vi "fiberphotometry_liveview.vi"() -> ()   [LabVIEW 2020]
uses:
  <userlib>/AndorSDK3/Data/GetPixelData16.vi
panel:
  in  "AOI Top":i64
  in  "AOI Left":i64
  in  "Binning":string
  in  "405 nm power (%)":i32
  in  "470 nm power (%)":i32
  in  "Apply Settings":bool
  in  "Centre AOI":bool
  in  "AOI Width":i64
  in  "AOI Height":i64
  out "Ready":bool
  in  "Run":bool
  in  "error":errorcluster
  out "Pixel Encoding":string
  out "Intensity Graph":u16[][](graph)
  out "AOIStride":i64
  out "PixelData":u16[](array[numeric])
  out "ByteData":u8[](array[numeric])
  in  "ExposureTime":dbl=0.1
  out "ImageSizeBytes":i64
  out "Handle":i32
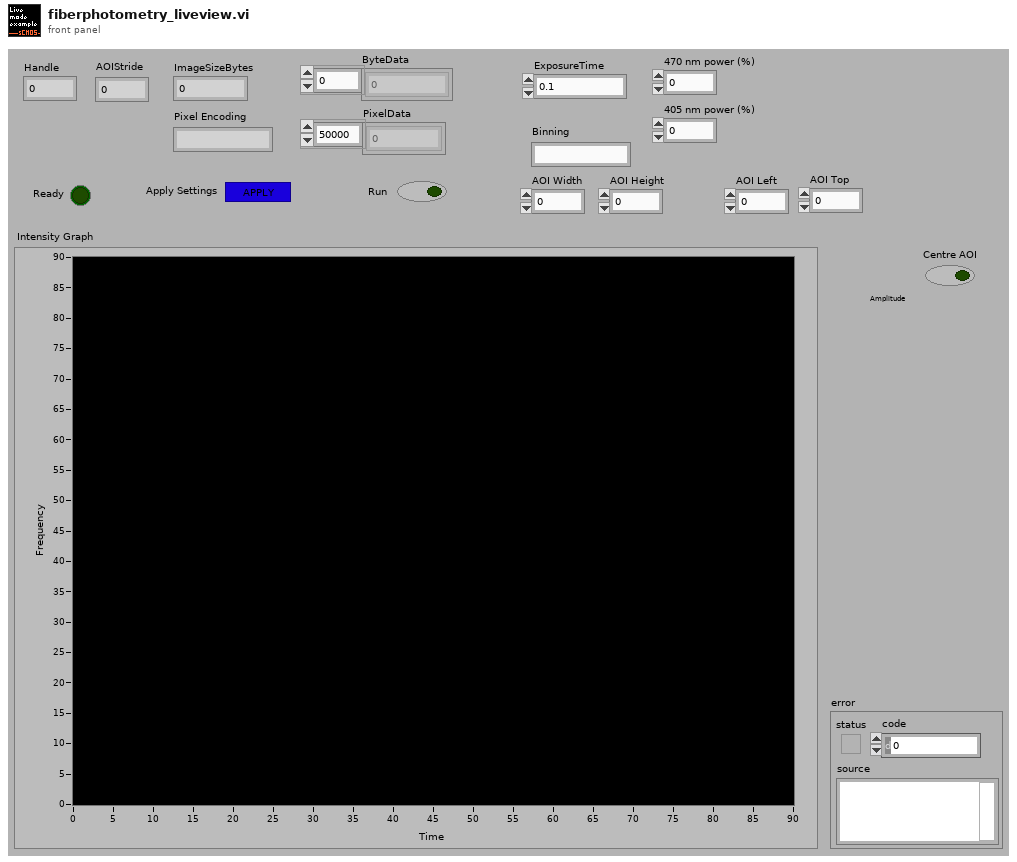
[diagram p1: front panel]
types:
  T1 = enum8{"Enabled", "Disabled", "Disabled and Grayed Out"}
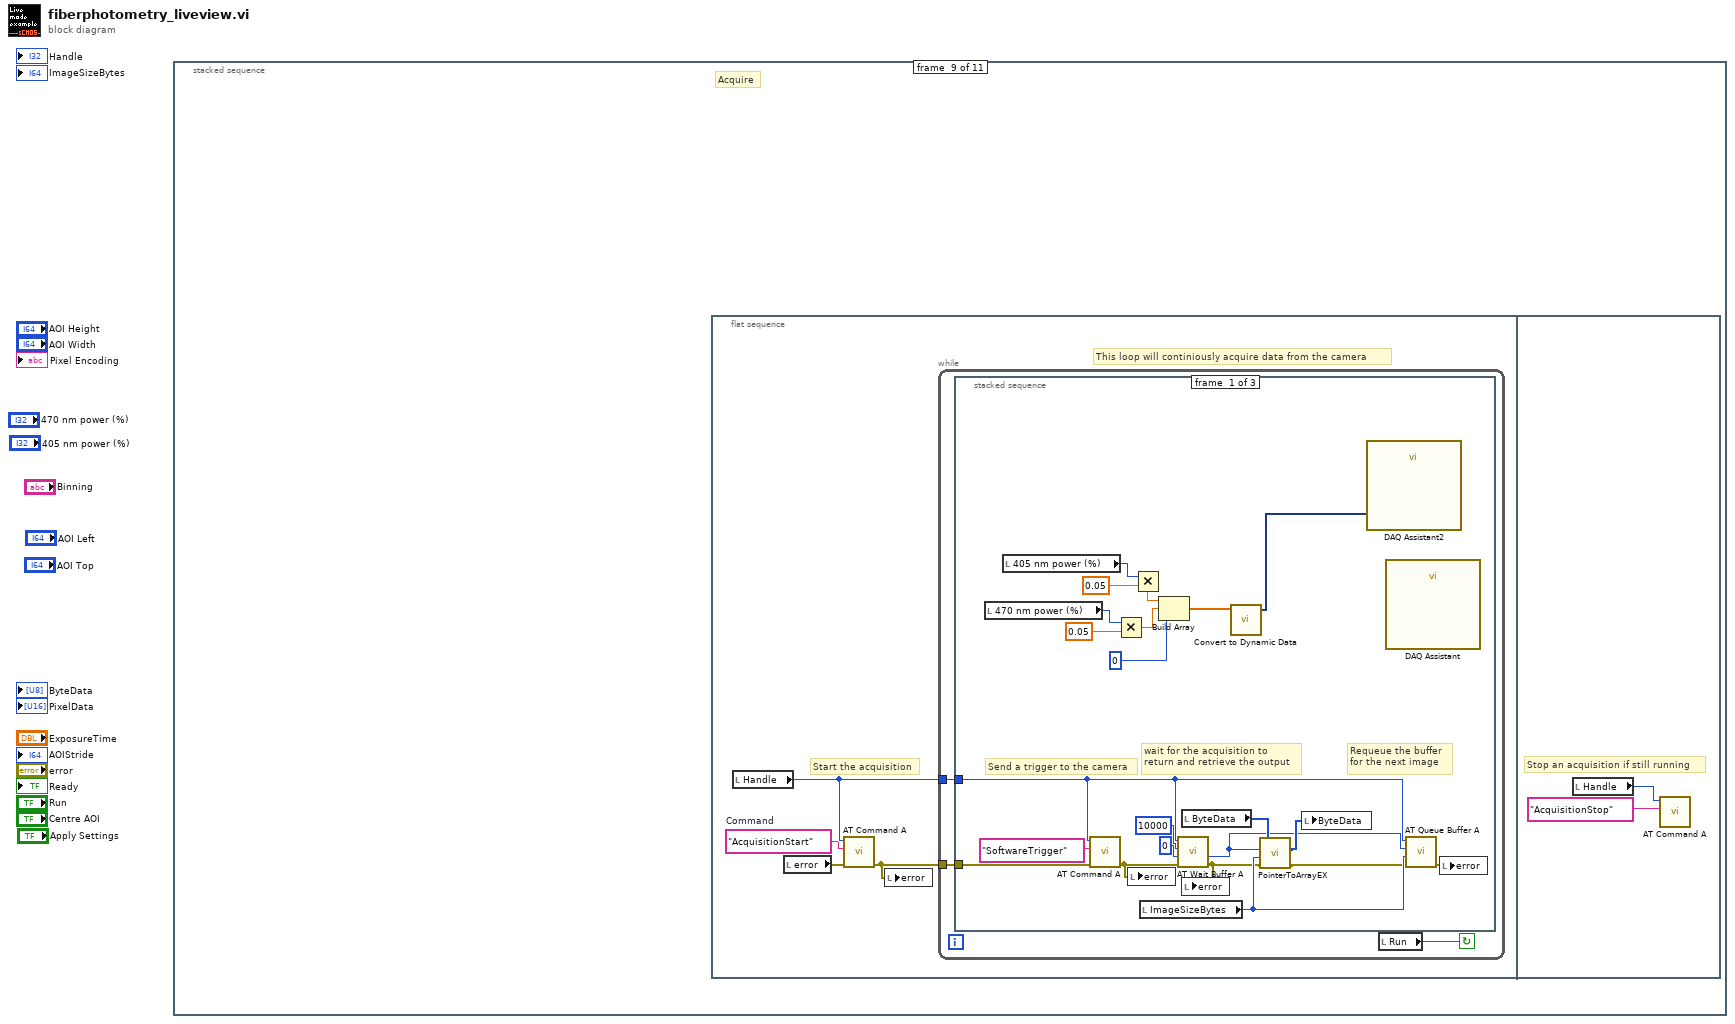
[diagram p0: block diagram]
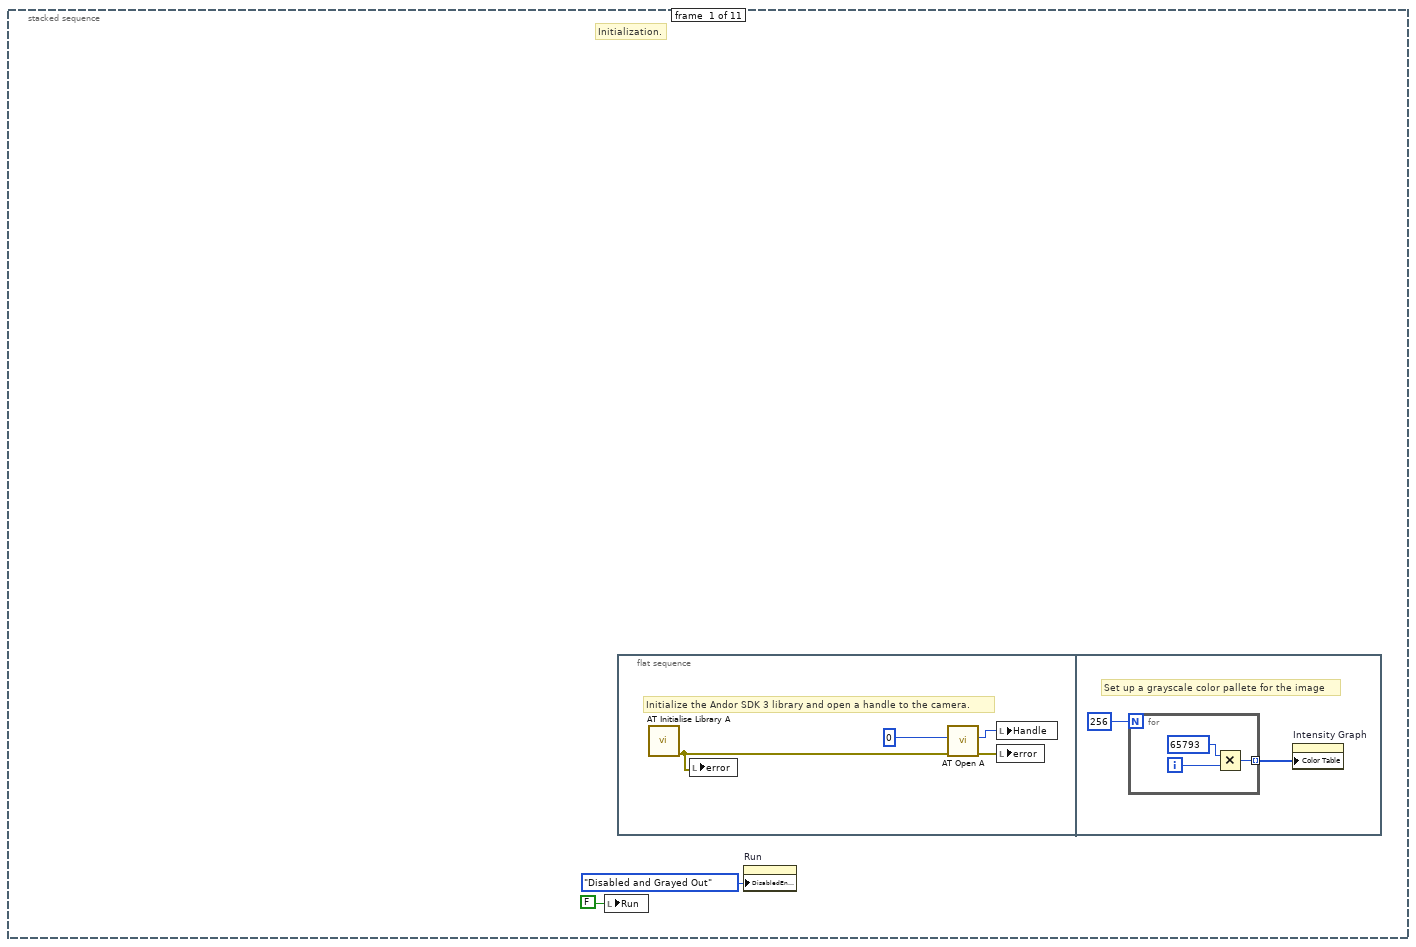
[diagram p2: hidden frame]
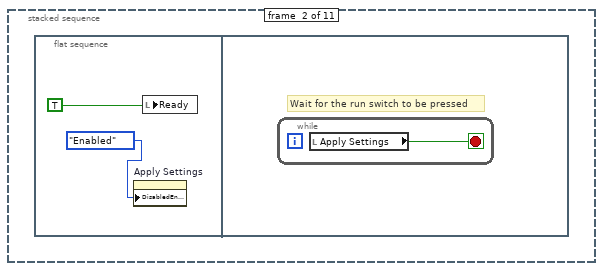
[diagram p3: hidden frame]
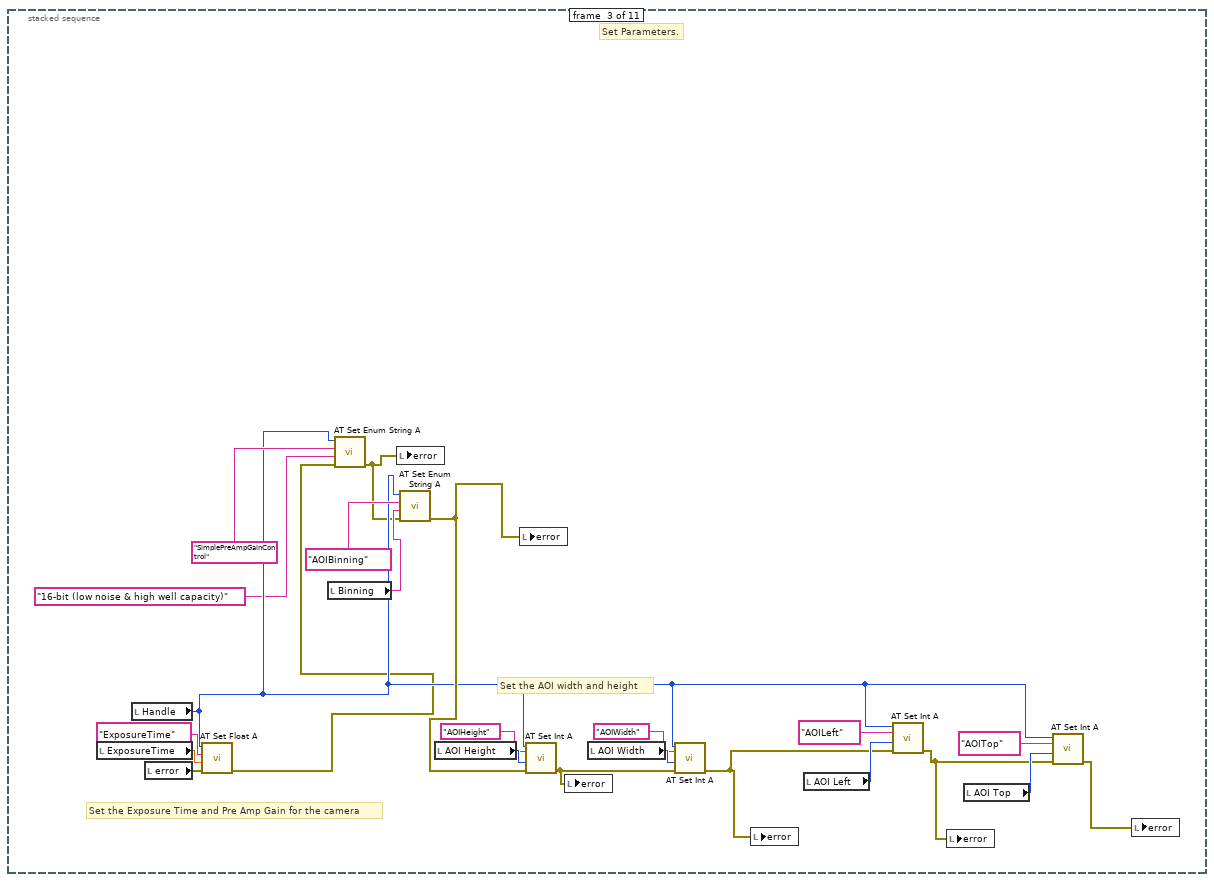
[diagram p4: hidden frame]
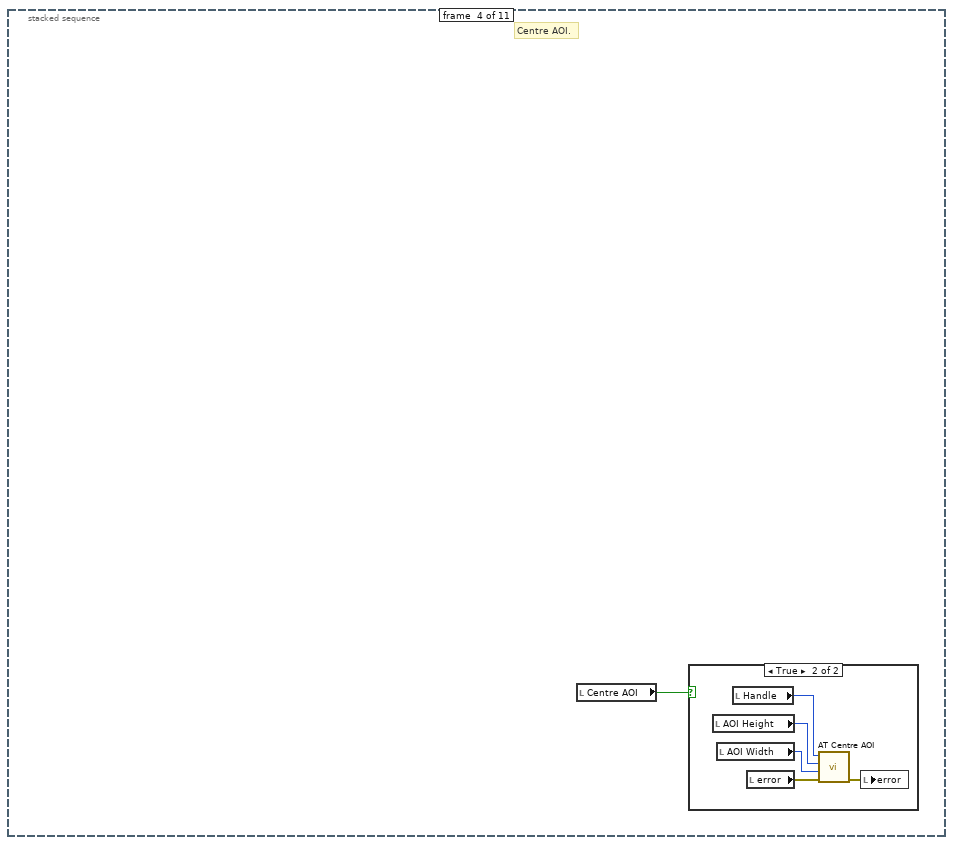
[diagram p5: hidden frame]
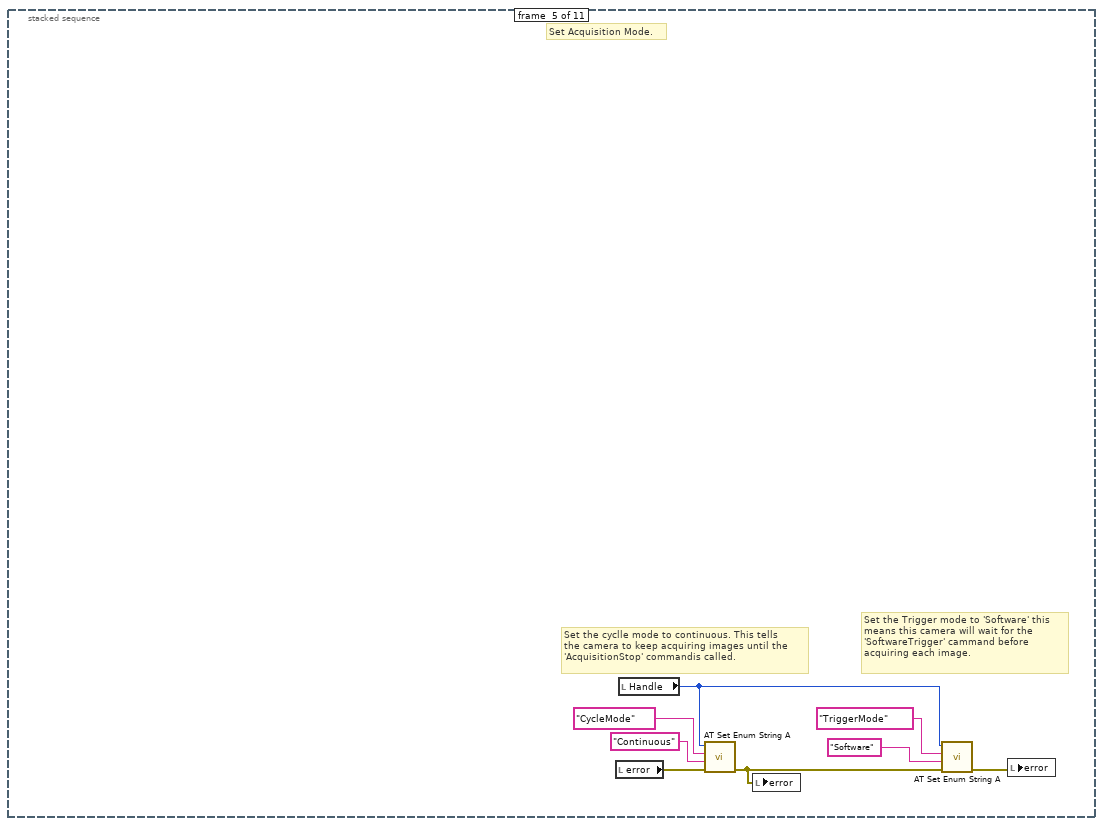
[diagram p7: hidden frame]
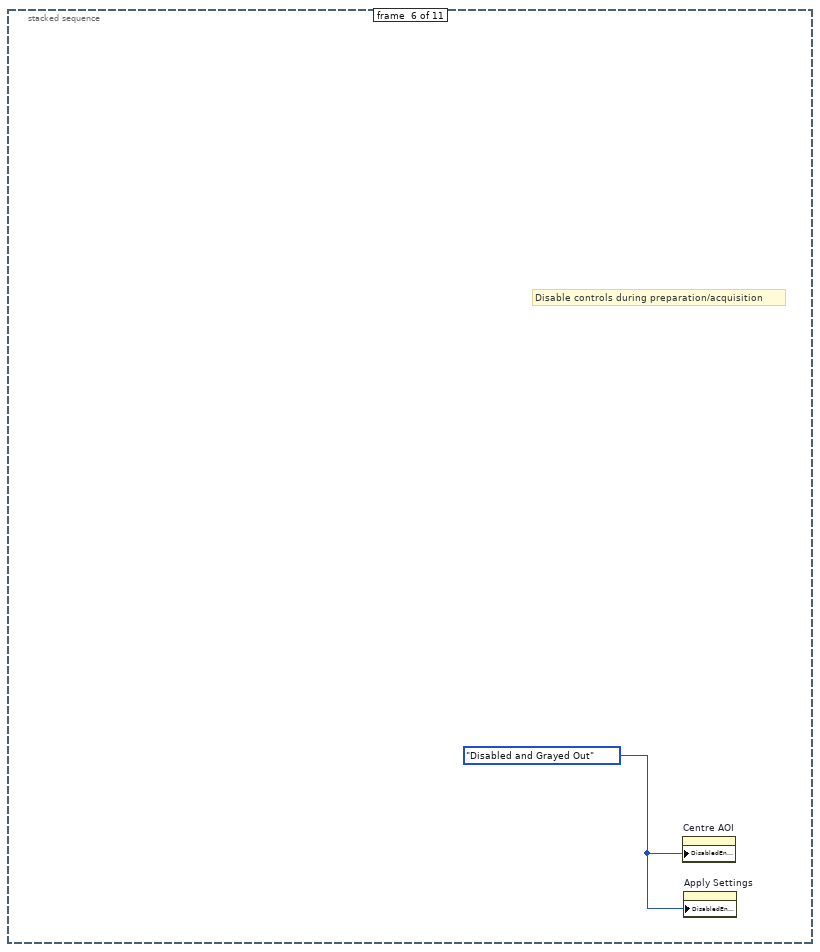
[diagram p8: hidden frame]
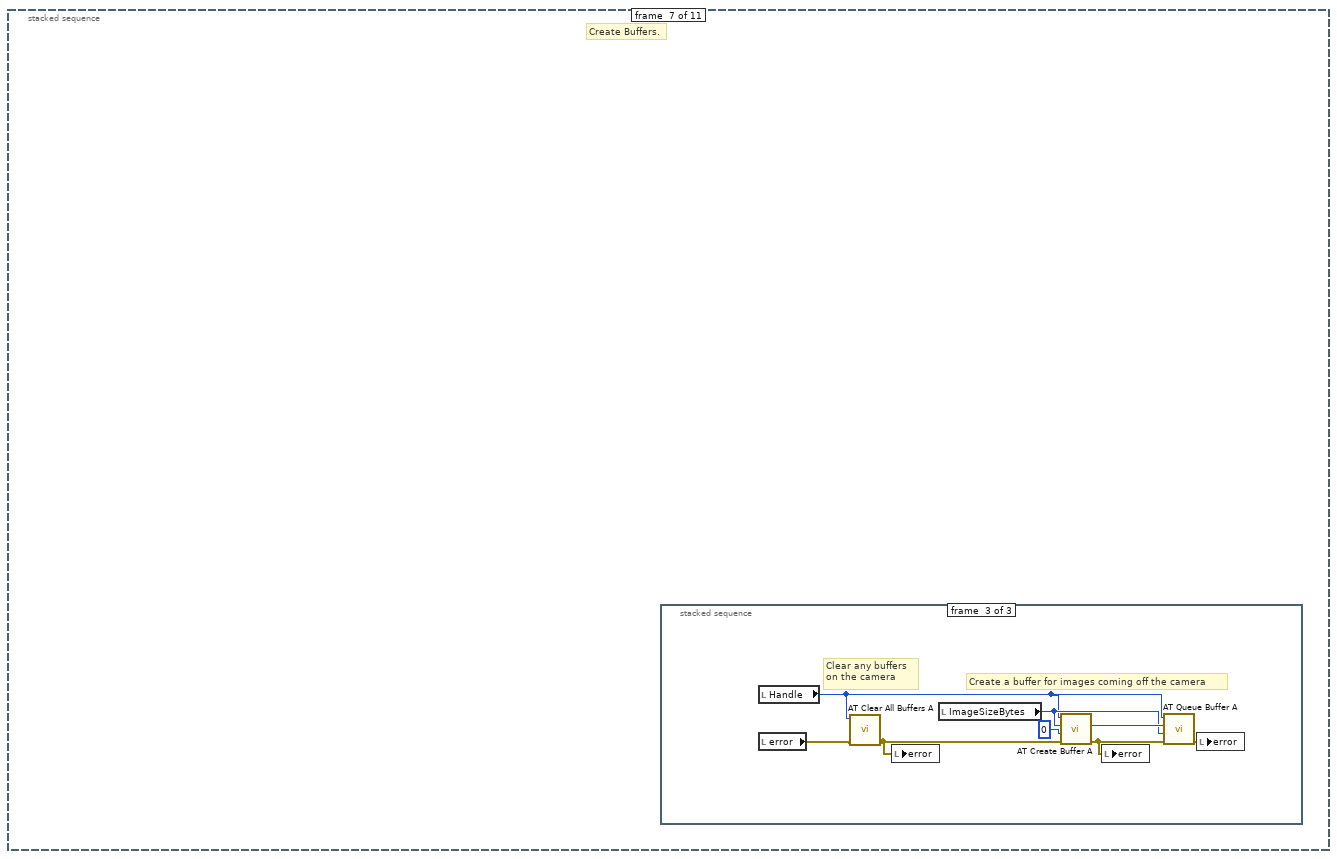
[diagram p9: hidden frame]
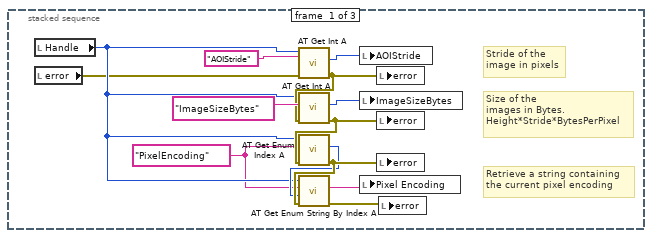
[diagram p10: hidden frame]
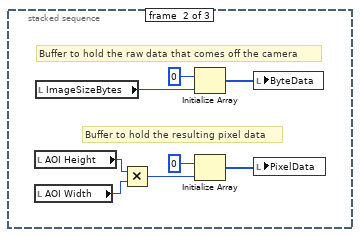
[diagram p11: hidden frame]
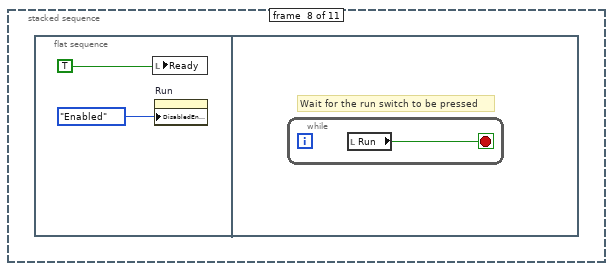
[diagram p12: hidden frame]
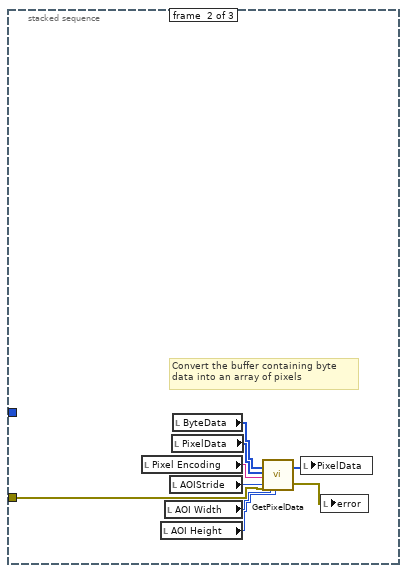
[diagram p13: hidden frame]
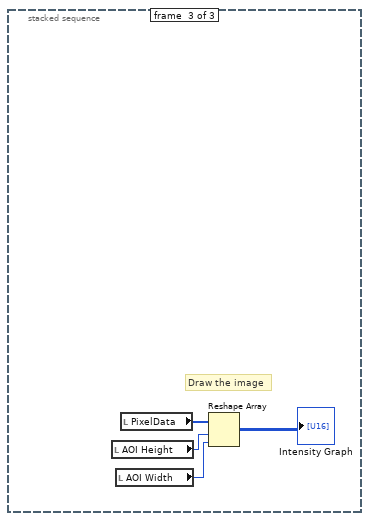
[diagram p14: hidden frame]
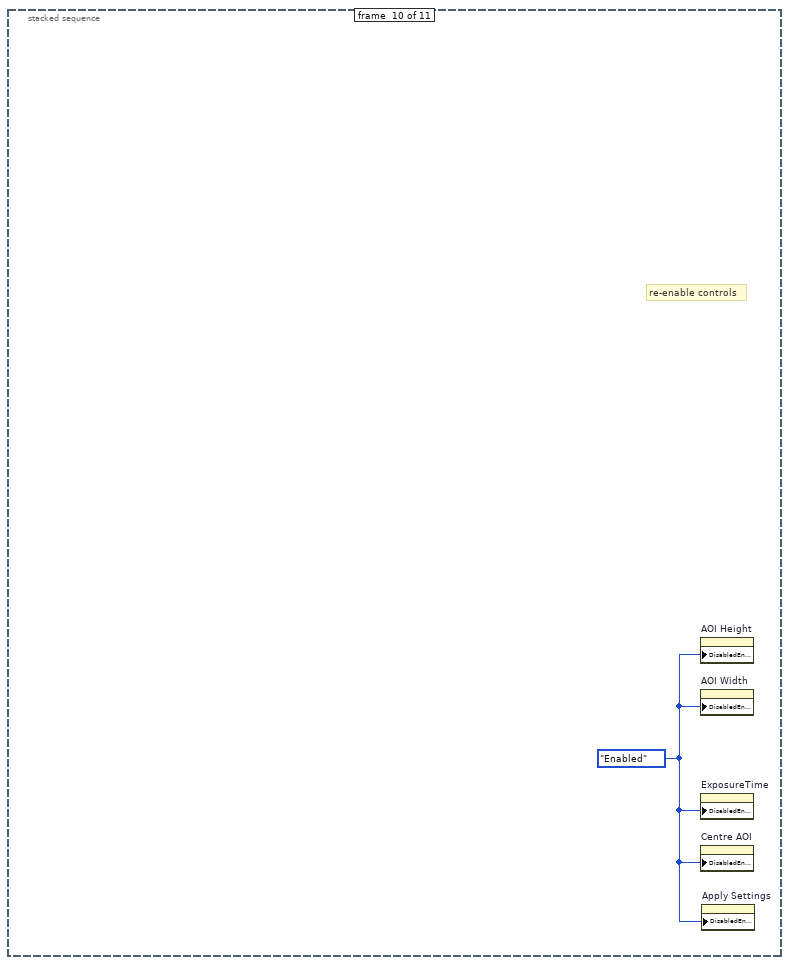
[diagram p15: hidden frame]
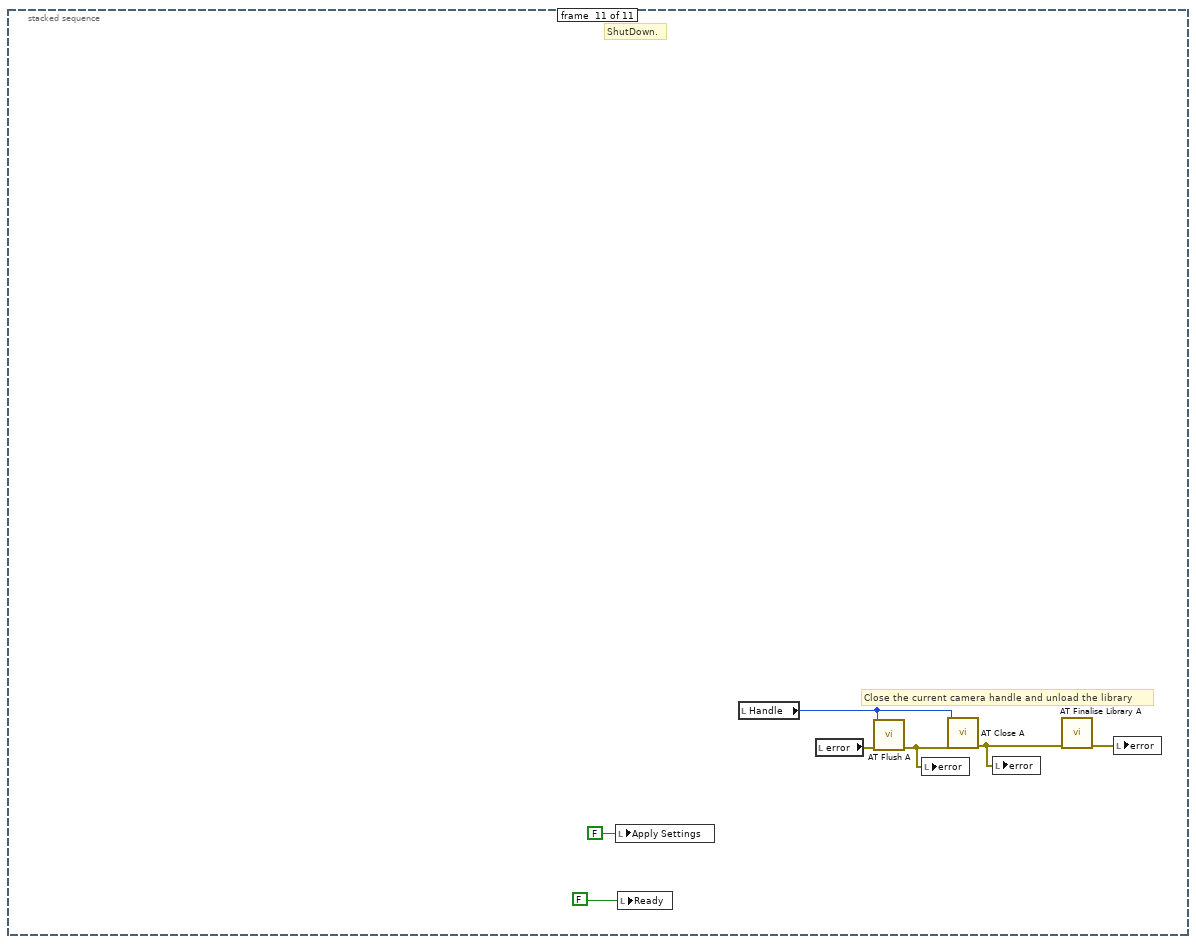
[diagram p16: hidden frame]
diagram:
  n1 = stacked-sequence {
    frame #0 {
      # "Initialization."
      n2 = local write "Run"(FALSE ("Run")) -> ()
      n3 = flat-sequence {
        frame #0 {
          # "Initialize the Andor SDK 3 library and open a handle to the camera."
          n4 = call <userlib>:"AT Initialise Library A.vi"() -> ("error out"=w4:errorcluster)  [unwired: 10 in, 1 out]
          n5 = local write "error"(w4) -> ()
          n6 = call <userlib>:"AT Open A.vi"("error in (no error)"=w4, "CameraIndex"=0) -> ("error out"=w3:errorcluster, "Handle"=w5:i32)  [unwired: 7 in, 1 out]
          n7 = local write "Handle"(w5) -> ()
          n8 = local write "error"(w3) -> ()
        }
        frame #1 {
          # "Set up a grayscale color pallete for the image"
          n9 = for {
            N: 256 -> [_]
            tunnel: [w10] -> w7 mode=indexing
            i -> [w11]
            n10 = Multiply(x=65793, y=w11) -> (x*y=w10:i32)
          }
          n11 = property on="Intensity Graph" class="IntGraph (strict)"("Color Table"=w7) -> ()  [unwired: 2 in, 2 out]
        }
      }
      n12 = property on="Run" class="Bool (strict)"("DisabledEnum"=T1."Disabled and Grayed Out" ("Disabled")) -> ()  [unwired: 2 in, 2 out]
    }
    frame #1 {
      n13 = flat-sequence {
        frame #0 {
          n14 = property on="Apply Settings" class="Bool (strict)"("DisabledEnum"=T1."Enabled" ("Disabled")) -> ()  [unwired: 2 in, 2 out]
          n15 = local write "Ready"(TRUE ("Ready")) -> ()
        }
        frame #1 {
          # "Wait for the run switch to be pressed"
          n16 = while {
            stop <- w14 stop-if-true
            n17 = local read "Apply Settings"() -> (w14:bool)
          }
        }
      }
    }
    frame #2 {
      # "Set the AOI width and height"
      # "Set the Exposure Time and Pre Amp Gain for the camera"
      # "Set Parameters."
      n18 = local read "ExposureTime"() -> (w37:dbl)
      n19 = local read "Handle"() -> (w18:i32)
      n20 = local read "error"() -> (w35:errorcluster)
      n21 = call <userlib>:"AT Set Float A.vi"("error in (no error)"=w35, "Value"=w37, "Feature"="ExposureTime" ("ExposureTime"), "Hndl"=w18) -> ("error out"=w17:errorcluster)  [unwired: 6 in, 1 out]
      n22 = local read "Binning"() -> (w28:string)
      n23 = call <userlib>:"AT Set Enum String A.vi"("error in (no error)"=w17, "String"="16-bit (low noise & high well capacity)", "Feature"="SimplePreAmpGainControl" ("Enum feature"), "Handle"=w18) -> ("error out"=w16:errorcluster)  [unwired: 6 in, 1 out]
      n24 = local write "error"(w16) -> ()
      n25 = call <userlib>:"AT Set Enum String A.vi"("error in (no error)"=w16, "String"=w28, "Feature"="AOIBinning" ("Enum feature"), "Handle"=w18) -> ("error out"=w27:errorcluster)  [unwired: 6 in, 1 out]
      n26 = local read "AOI Height"() -> (w33:i64)
      n27 = local write "error"(w27) -> ()
      n28 = call <userlib>:"AT Set Int A.vi"("error in (no error)"=w27, "Value"=w33, "Feature"="AOIHeight" ("Integer feature"), "Handle"=w18) -> ("error out"=w34:errorcluster)  [unwired: 6 in, 1 out]
      n29 = local write "error"(w34) -> ()
      n30 = local read "AOI Width"() -> (w32:i64)
      n31 = call <userlib>:"AT Set Int A.vi"("error in (no error)"=w34, "Value"=w32, "Feature"="AOIWidth" ("Integer feature 2"), "Handle"=w18) -> ("error out"=w22:errorcluster)  [unwired: 6 in, 1 out]
      n32 = local write "error"(w22) -> ()
      n33 = local read "AOI Left"() -> (w26:i64)
      n34 = call <userlib>:"AT Set Int A.vi"("error in (no error)"=w22, "Value"=w26, "Feature"="AOILeft" ("Integer feature 2"), "Handle"=w18) -> ("error out"=w21:errorcluster)  [unwired: 6 in, 1 out]
      n35 = local write "error"(w21) -> ()
      n36 = local read "AOI Top"() -> (w24:i64)
      n37 = call <userlib>:"AT Set Int A.vi"("error in (no error)"=w21, "Value"=w24, "Feature"="AOITop" ("Integer feature 2"), "Handle"=w18) -> ("error out"=w20:errorcluster)  [unwired: 6 in, 1 out]
      n38 = local write "error"(w20) -> ()
    }
    frame #3 {
      # "Centre AOI."
      n39 = local read "Centre AOI"() -> (w38:bool)
      n40 = case shown="True" w38 {
        frame False {
        }
        frame True {
          n41 = local read "AOI Height"() -> (w40:i64)
          n42 = local read "AOI Width"() -> (w41:i64)
          n43 = local read "Handle"() -> (w39:i32)
          n44 = local read "error"() -> (w42:errorcluster)
          n45 = call <userlib>:"AT Centre AOI.vi"("error in (no error)"=w42, "AOI Width"=w41, "AOI Height"=w40, "Handle"=w39) -> ("error out"=w43:errorcluster)  [unwired: 7 in]
          n46 = local write "error"(w43) -> ()
        }
      }
    }
    frame #4 {
      # "Set the Trigger mode to 'Software' this \nmeans this camera will wait for the \n'SoftwareTrigger' cammand before \nacquiring each image."
      # "Set the cyclle mode to continuous. This tells \nthe camera to keep acquiring images until the \n'AcquisitionStop' commandis called."
      # "Set Acquisition Mode."
      n47 = local read "error"() -> (w50:errorcluster)
      n48 = local read "Handle"() -> (w48:i32)
      n49 = call <userlib>:"AT Set Enum String A.vi"("error in (no error)"=w50, "String"="Continuous", "Feature"="CycleMode" ("Enum feature"), "Handle"=w48) -> ("error out"=w49:errorcluster)  [unwired: 6 in, 1 out]
      n50 = local write "error"(w49) -> ()
      n51 = call <userlib>:"AT Set Enum String A.vi"("error in (no error)"=w49, "String"="Software", "Feature"="TriggerMode" ("Enum feature"), "Handle"=w48) -> ("error out"=w46:errorcluster)  [unwired: 6 in, 1 out]
      n52 = local write "error"(w46) -> ()
    }
    frame #5 {
      w52 = T1."Disabled and Grayed Out" ("Disabled")
      # "Disable controls during preparation/acquisition"
      n53 = property on="Centre AOI" class="Bool (strict)"("DisabledEnum"=w52) -> ()  [unwired: 2 in, 2 out]
      n54 = property on="Apply Settings" class="Bool (strict)"("DisabledEnum"=w52) -> ()  [unwired: 2 in, 2 out]
    }
    frame #6 {
      # "Create Buffers."
      n55 = stacked-sequence {
        frame #0 {
          w53 = "PixelEncoding" ("Enum feature")
          # "Retrieve a string containing \nthe current pixel encoding"
          # "Stride of the\nimage in pixels"
          # "Size of the\nimages in Bytes.\nHeight*Stride*BytesPerPixel"
          n56 = local read "Handle"() -> (w55:i32)
          n57 = local read "error"() -> (w54:errorcluster)
          n58 = call <userlib>:"AT Get Int A.vi"("error in (no error)"=w54, "Feature"="AOIStride" ("Integer feature"), "Handle"=w55) -> ("error out"=w61:errorcluster, "Value"=w65:i64)  [unwired: 6 in, 1 out]
          n59 = call <userlib>:"AT Get Int A.vi"("error in (no error)"=w61, "Feature"="ImageSizeBytes" ("Integer feature"), "Handle"=w55) -> ("error out"=w60:errorcluster, "Value"=w64:i64)  [unwired: 6 in, 1 out]
          n60 = call <userlib>:"AT Get Enum Index A.vi"("error in (no error)"=w60, "Feature"=w53, "Handle"=w55) -> ("error out"=w59:errorcluster, "Value"=w58:i32)  [unwired: 6 in, 1 out]
          n61 = call <userlib>:"AT Get Enum String By Index A.vi"("error in (no error)"=w59, "Index"=w58, "Feature"=w53, "Handle"=w55) -> ("error out"=w56:errorcluster, "String"=w57:string)  [unwired: 5 in, 1 out]
          n62 = local write "AOIStride"(w65) -> ()
          n63 = local write "ImageSizeBytes"(w64) -> ()
          n64 = local write "Pixel Encoding"(w57) -> ()
          n65 = local write "error"(w61) -> ()
          n66 = local write "error"(w60) -> ()
          n67 = local write "error"(w59) -> ()
          n68 = local write "error"(w56) -> ()
        }
        frame #1 {
          # "Buffer to hold the resulting pixel data"
          # "Buffer to hold the raw data that comes off the camera"
          n69 = local read "AOI Height"() -> (w71:i64)
          n70 = local read "AOI Width"() -> (w72:i64)
          n71 = local read "ImageSizeBytes"() -> (w67:i64)
          n72 = Multiply(x=w71, y=w72) -> (x*y=w66:i64)
          n73 = Initialize Array(u8 0, w67) -> (w69:u8[])
          n74 = Initialize Array(i64 0, w66) -> (w70:i64[])
          n75 = local write "ByteData"(w69) -> ()
          n76 = local write "PixelData"(w70) -> ()
        }
        frame #2 {
          # "Clear any buffers \non the camera"
          # "Create a buffer for images coming off the camera"
          n77 = local read "Handle"() -> (w74:i32)
          n78 = local read "error"() -> (w76:errorcluster)
          n79 = call <userlib>:"AT Clear All Buffers A.vi"("error in (no error)"=w76, "Handle"=w74) -> ("error out"=w75:errorcluster)  [unwired: 8 in, 1 out]
          n80 = local write "error"(w75) -> ()
          n81 = local read "ImageSizeBytes"() -> (w78:i64)
          n82 = call <userlib>:"AT Create Buffer A.vi"("error in (no error)"=w75, "Buffer"=0 ("Size"), "Size"=w78, "Handle"=w74) -> ("error out"=w80:errorcluster, "Buffer out"=w81:u64)  [unwired: 5 in, 1 out]
          n83 = local write "error"(w80) -> ()
          n84 = call <userlib>:"AT Queue Buffer A.vi"("error in (no error)"=w80, "PtrSize"=w78, "Ptr"=w81, "Handle"=w74) -> ("error out"=w77:errorcluster)  [unwired: 6 in, 1 out]
          n85 = local write "error"(w77) -> ()
        }
      }
    }
    frame #7 {
      n86 = flat-sequence {
        frame #0 {
          n87 = local write "Ready"(TRUE ("Ready")) -> ()
          n88 = property on="Run" class="Bool (strict)"("DisabledEnum"=T1."Enabled" ("Disabled")) -> ()  [unwired: 2 in, 2 out]
        }
        frame #1 {
          # "Wait for the run switch to be pressed"
          n89 = while {
            stop <- w84 stop-if-true
            n90 = local read "Run"() -> (w84:bool)
          }
        }
      }
    }
    frame #8 {
      # "Acquire"
      n91 = flat-sequence {
        frame #0 {
          w86 = "AcquisitionStart"  # Command
          # "This loop will continiously acquire data from the camera"
          # "Start the acquisition"
          n92 = local read "Handle"() -> (w88:i32)
          n93 = local read "error"() -> (w87:errorcluster)
          n94 = call <userlib>:"AT Command A.vi"("error in (no error)"=w87, "Feature"=w86, "Handle"=w88) -> ("error out"=w85:errorcluster)  [unwired: 7 in, 1 out]
          n95 = local write "error"(w85) -> ()
          n96 = while {
            tunnel: w88 -> [w90]
            tunnel: w85 -> [w91]
            stop <- w89 continue-if-true
            n97 = stacked-sequence {
              tunnel: w91 -> [w108 w114 _]
              tunnel: w90 -> [w109 _ _]
              frame #0 {
                # "Requeue the buffer\nfor the next image"
                # "Send a trigger to the camera"
                # "wait for the acquisition to \nreturn and retrieve the output"
                n98 = local read "470 nm power (%)"() -> (w94:i32)
                n99 = local read "405 nm power (%)"() -> (w93:i32)
                n100 = call <userlib>:"AT Command A.vi"("error in (no error)"=w108, "Feature"="SoftwareTrigger" ("Command"), "Handle"=w109) -> ("error out"=w107:errorcluster)  [unwired: 7 in, 1 out]
                n101 = Multiply(x=w94, y=0.05) -> (x*y=w95:dbl)
                n102 = local write "error"(w107) -> ()
                n103 = Multiply(x=w93, y=0.05) -> (x*y=w100:dbl)
                n104 = local read "ImageSizeBytes"() -> (w105:i64)
                n105 = Build Array(w100, w95, 0) -> (w97:dbl[])
                n106 = call <userlib>:"AT Wait Buffer A.vi"("error in (no error)"=w107, "Input buffer"=u32 0, "Timeout"=u32 10000, "Handle"=w109) -> ("error out"=w102:errorcluster, "Output buffer"=w101:u64)  [unwired: 4 in, 2 out]
                n107 = local read "ByteData"() -> (w106:u8[])
                n108 = local write "error"(w102) -> ()
                n109 = call "Convert to Dynamic Data"("Array"=w97) -> ("Dynamic Data Type"=w92:dynamicdata)  [unwired: 3 in]
                n110 = call <userlib>:"PointerToArrayEX.vi"("Array in"=w106, "Pointer In"=w101, "Pointer Size"=w105, "error in (no error)"=w102) -> ("Array out"=w104:u8[], "error out"=w103:errorcluster)  [unwired: 4 in]
                n111 = local write "ByteData"(w104) -> ()
                n112 = call "DAQ Assistant2"("data"=w92) -> ()  [unwired: 17 in, 2 out]
                n113 = call "DAQ Assistant"() -> ()  [unwired: 18 in, 2 out]
                n114 = call <userlib>:"AT Queue Buffer A.vi"("error in (no error)"=w103, "PtrSize"=w105, "Ptr"=w101, "Handle"=w109) -> ("error out"=w111:errorcluster)  [unwired: 6 in, 1 out]
                n115 = local write "error"(w111) -> ()
              }
              frame #1 {
                # "Convert the buffer containing byte \ndata into an array of pixels"
                n116 = local read "Pixel Encoding"() -> (w120:string)
                n117 = local read "AOI Height"() -> (w117:i64)
                n118 = local read "AOI Width"() -> (w118:i64)
                n119 = local read "AOIStride"() -> (w121:i64)
                n120 = local read "PixelData"() -> (w119:u16[])
                n121 = local read "ByteData"() -> (w115:u8[])
                n122 = call-poly <userlib>:"GetPixelData.vi"("Input buffer"=w115, "Output buffer in"=w119, "Pixel Encoding"=w120, "Stride"=w121, "error in (no error)"=w114, "Width"=w118, "Height"=w117) -> ("Output buffer out"=w122:u16[], "error out"=w116:errorcluster)  [unwired: 10 in, 1 out]
                n123 = local write "PixelData"(w122) -> ()
                n124 = local write "error"(w116) -> ()
              }
              frame #2 {
                # "Draw the image"
                n125 = local read "AOI Height"() -> (w125:i64)
                n126 = local read "AOI Width"() -> (w124:i64)
                n127 = local read "PixelData"() -> (w126:u16[])
                n128 = Reshape Array(w126, w125, w124) -> (→"Intensity Graph":u16[][])
              }
            }
            n129 = local read "Run"() -> (w89:bool)
          }
        }
        frame #1 {
          # "Stop an acquisition if still running"
          n130 = local read "Handle"() -> (w128:i32)
          n131 = call <userlib>:"AT Command A.vi"("Feature"="AcquisitionStop" ("Command"), "Handle"=w128) -> ()  [unwired: 8 in, 2 out]
        }
      }
    }
    frame #9 {
      w129 = T1."Enabled" ("Disabled")
      # "re-enable controls"
      n132 = property on="AOI Height" class="DigNum (strict)"("DisabledEnum"=w129) -> ()  [unwired: 2 in, 2 out]
      n133 = property on="AOI Width" class="DigNum (strict)"("DisabledEnum"=w129) -> ()  [unwired: 2 in, 2 out]
      n134 = property on="ExposureTime" class="DigNum (strict)"("DisabledEnum"=w129) -> ()  [unwired: 2 in, 2 out]
      n135 = property on="Centre AOI" class="Bool (strict)"("DisabledEnum"=w129) -> ()  [unwired: 2 in, 2 out]
      n136 = property on="Apply Settings" class="Bool (strict)"("DisabledEnum"=w129) -> ()  [unwired: 2 in, 2 out]
    }
    frame #10 {
      # "Close the current camera handle and unload the library"
      # "ShutDown."
      n137 = local write "Apply Settings"(FALSE ("Apply Settings")) -> ()
      n138 = local write "Ready"(FALSE ("Ready")) -> ()
      n139 = local read "Handle"() -> (w132:i32)
      n140 = local read "error"() -> (w134:errorcluster)
      n141 = call <userlib>:"AT Flush A.vi"("error in (no error)"=w134, "Handle"=w132) -> ("error out"=w135:errorcluster)  [unwired: 8 in, 1 out]
      n142 = local write "error"(w135) -> ()
      n143 = call <userlib>:"AT Close A.vi"("error in (no error)"=w135, "Handle"=w132) -> ("error out"=w136:errorcluster)  [unwired: 8 in, 1 out]
      n144 = local write "error"(w136) -> ()
      n145 = call <userlib>:"AT Finalise Library A.vi"("error in (no error)"=w136) -> ("error out"=w133:errorcluster)  [unwired: 9 in, 1 out]
      n146 = local write "error"(w133) -> ()
    }
  }
